vi "Dequeue Element.vi"(8 "error in (no error)":errorcluster, 9 "timeout in ms (10)":i32=10, 11 "QDMH in":refnum<class "QDMH.lvclass">) -> (0 "error out":errorcluster, 1 "State":string, 2 "Data":variant, 3 "QDMH out":refnum<class "QDMH.lvclass">, 4 "Remaining":i32)   [LabVIEW 2023, in "QDMH.lvlib" / "QDMH.lvclass"]
doc: "This VI dequeues the next element in the queue. Additionally, it checks the status of the queue to see how many elements are unprocessed in the queue. This is for monitoring purposes and should be used to identify when the queue is filling up faster than it can process."
uses:
  QDMH.lvclass
  QDMH.lvclass/QDMH.ctl
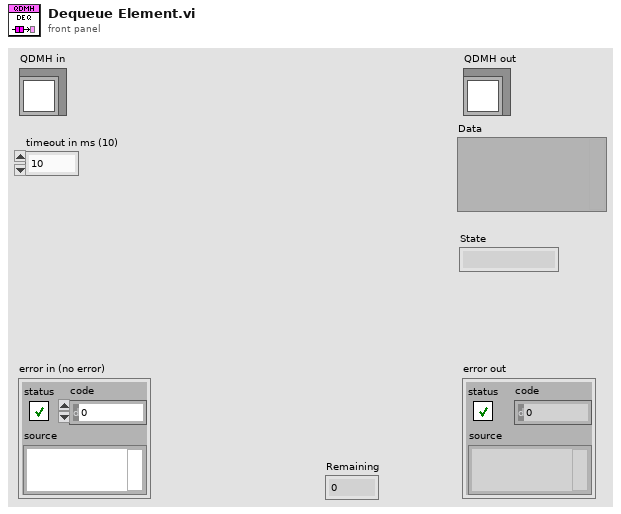
[diagram p1: front panel]
types:
  T1 = typedef "QDMH.lvlib/QDMH.lvclass/QDMH Message.ctl" = cluster{"State":string, "Data":variant}
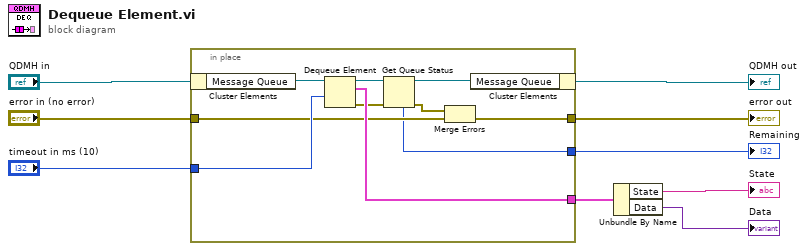
[diagram p0: block diagram]
diagram:
  n1 = in-place {
    in-place-border: [w17] -> w4
    in-place-border: "error in (no error)" -> [w15]
    in-place-border: "timeout in ms (10)" -> [w16]
    in-place-border: [w12] -> w5
    in-place-border: [w13] -> w1
    n2 = in-place-cluster #1("QDMH in") -> ("Message Queue"=w19:refnum<queue>)
    n3 = Dequeue Element(queue=w19, timeout in ms (-1)=w16) -> (queue out=w18:refnum<queue>, element=w17:T1, error out=w11:errorcluster)  [unwired: 1 in, 1 out]
    n4 = Get Queue Status(queue=w18, error in (no error)=w11) -> (queue out=w14:refnum<queue>, error out=w10:errorcluster, # elements in queue=w13:i32)  [unwired: 1 in, 5 out]
    n5 = Merge Errors(w10, w15) -> (w12:errorcluster)
    n6 = in-place-cluster #1("Message Queue"=w14) -> (→"QDMH out":refnum<class "QDMH.lvclass">)
  }
  "error out" <- w5
  "Remaining" <- w1
  n7 = Unbundle By Name(w4) -> ("State"=→"State":string, "Data"=→"Data":variant)
